vi "dfd_Build Remez Band Parameter from Classical Filter Specs.vi"(6 "fs [Hz]":dbl=1.0 format="%.2f", 7 "filter type":T4(ring), 8 "error in (no error)":errorcluster, 10 "ripple specs":T1={"passband"=0.1, "stopband"=60.0, "dB/linear? (T: dB)"=TRUE}, 11 "freq specs [Hz]":T3) -> (0 "error out":errorcluster, 1 "band ripples":dbl[](array[numeric]), 2 "band parameters":T2[](array[typedef])=[{"band specification"=[{"freq"=0.0, "amplitude"=1.0, "weight"=1.0}, {"freq"=0.2, "amplitude"=1.0, "weight"=1.0}], "ripple constraint"=0.0}, {"band specification"=[{"freq"=0.3, "amplitude"=0.0, "weight"=1.0}, {"freq"=0.5, "amplitude"=0.0, "weight"=1.0}], "ripple constraint"=0.0}])   [LabVIEW 2017, in "NI_DigFilterLicensed.lvlib"]
uses:
  <vilib>/addons/Digital Filter Design/NI_DigFilterLicensed.lvlib
  <vilib>/addons/Digital Filter Design/_Objects.llb/DFD Filter Frequence Specification (Design).ctl
  <vilib>/addons/Digital Filter Design/_Objects.llb/DFD Adv Band Spec.ctl
  <vilib>/addons/Digital Filter Design/_Objects.llb/DFD Filter Ripple Specification (Design).ctl
  <vilib>/addons/Digital Filter Design/NI_DigFilter_Design.lvlib
panel:
  # "freq"
  # "amplitude"
  # "weight"
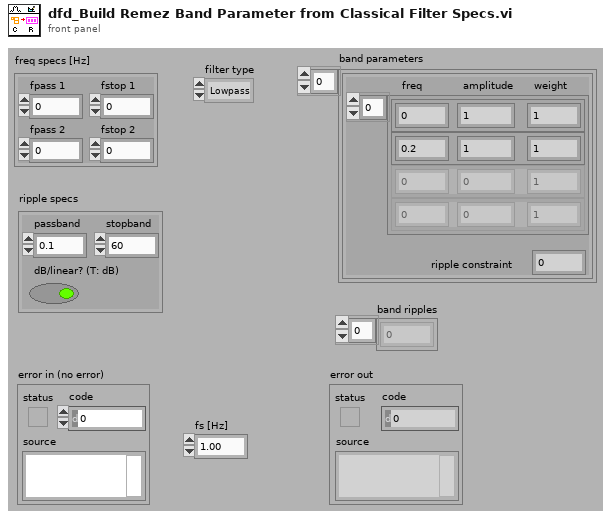
[diagram p1: front panel]
types:
  T1 = typedef "NI_DigFilterLicensed.lvlib/DFD Filter Ripple Specification (Design).ctl" = cluster{"passband":dbl, "stopband":dbl, "dB/linear? (T: dB)":bool}
  T2 = typedef "NI_DigFilterLicensed.lvlib/DFD Adv Band Spec.ctl" = cluster{"band specification":cluster{"freq":dbl, "amplitude":dbl, "weight":dbl}[], "ripple constraint":dbl}
  T3 = typedef "NI_DigFilterLicensed.lvlib/DFD Filter Frequence Specification (Design).ctl" = cluster{"fpass 1":dbl, "fstop 1":dbl, "fpass 2 ":dbl, "fstop 2":dbl}
  T4 = enum16{"Lowpass", "Highpass", "Bandpass", "Bandstop"}
  T5 = cluster{cluster{"fpass 1":dbl, dbl, "stopband":dbl}[], "passband":dbl}
  T6 = cluster{cluster{"fstop 1":dbl, dbl, "passband":dbl}[], "stopband":dbl}
  T7 = cluster{cluster{"fstop 1":dbl, dbl, "passband":dbl}[], "stopband":dbl}[]
  T8 = cluster{cluster{"fpass 1":dbl, dbl, "stopband":dbl}[], "passband":dbl}[]
  T9 = cluster{cluster{"fpass 2 ":dbl, dbl, "stopband":dbl}[], "passband":dbl}
  T10 = cluster{cluster{"fstop 2":dbl, dbl, "passband":dbl}[], "stopband":dbl}
  T11 = cluster{cluster{"fstop 2":dbl, dbl, "passband":dbl}[], "stopband":dbl}[]
  T12 = cluster{cluster{"fpass 2 ":dbl, dbl, "stopband":dbl}[], "passband":dbl}[]
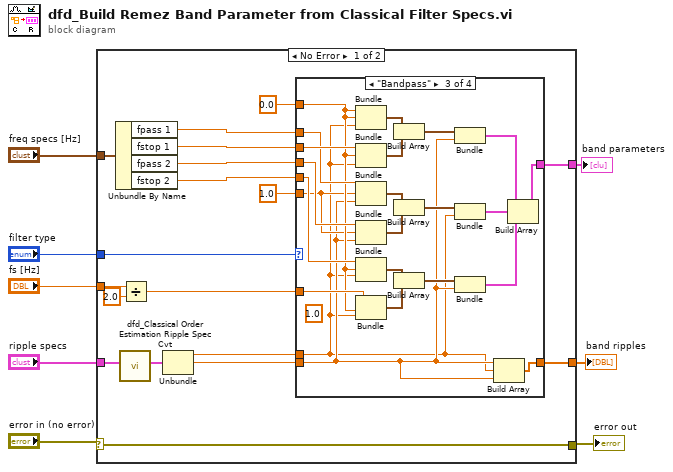
[diagram p0: block diagram]
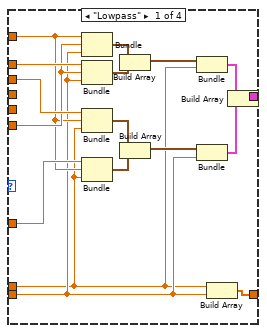
[diagram p2: hidden frame]
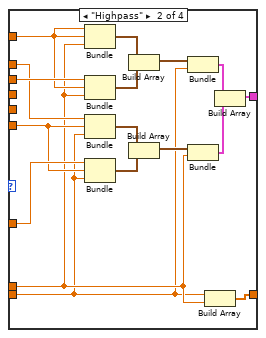
[diagram p3: hidden frame]
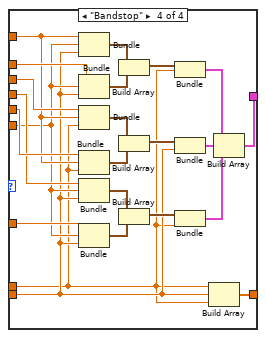
[diagram p4: hidden frame]
diagram:
  n1 = case shown="No Error" "error in (no error)" {
    selector: "error in (no error)" -> [w16 w107]
    tunnel: "filter type" -> [w26 _]
    tunnel: "freq specs [Hz]" -> [w25 _]
    tunnel: [w24 _] -> w6
    tunnel: "fs [Hz]" -> [w19 _]
    tunnel: "ripple specs" -> [w15 _]
    tunnel: [w16 w107] -> w2
    tunnel: [w14 _] -> w1
    frame No Error {
      n2 = Unbundle By Name(w25) -> ("fpass 1"=w23:dbl, "fstop 1"=w22:dbl, "fpass 2"=w21:dbl, "fstop 2"=w20:dbl)
      n3 = call <vilib>:"dfd_Classical Order Estimation Ripple Spec Cvt.vi"("ripple specs"=w15) -> ("ripple specs (linear)"=w13:T1)  [unwired: 10 out]
      n4 = Divide(x=w19, y=2.0) -> (x/y=w17:dbl)
      n5 = Unbundle(w13) -> ("passband"=w12:dbl, "stopband"=w11:dbl)  [unwired: 1 out]
      n6 = case shown="\"Bandpass\"" w26 {
        tunnel: w23 -> [w41 w54 w71 w95]
        tunnel: w22 -> [w35 w55 w72 w94]
        tunnel: w21 -> [_ _ w70 w92]
        tunnel: w20 -> [_ _ w69 w93]
        tunnel: [w34 w51 w67 w90] -> w24
        tunnel: w17 -> [w32 w49 w66 w89]
        tunnel: [w31 w48 w65 w88] -> w14
        tunnel: w12 -> [w27 w45 w61 w84]
        tunnel: w11 -> [w28 w44 w62 w85]
        tunnel: 0.0 -> [w29 w46 w64 w87]
        tunnel: 1.0 -> [w30 w47 w63 w86]
        frame "Lowpass" {
          n7 = Bundle(w29, w30, "stopband"=w28) -> (w43:cluster{dbl, dbl, "stopband":dbl})  [unwired: 1 out]
          n8 = Bundle("fpass 1"=w41, w30, "stopband"=w28) -> (w42:cluster{"fpass 1":dbl, dbl, "stopband":dbl})  [unwired: 1 out]
          n9 = Bundle("fstop 1"=w35, w29, "passband"=w27) -> (w37:cluster{"fstop 1":dbl, dbl, "passband":dbl})  [unwired: 1 out]
          n10 = Bundle(w32, w29, "passband"=w27) -> (w38:cluster{dbl, dbl, "passband":dbl})  [unwired: 1 out]
          n11 = Build Array(w43, w42) -> (w40:cluster{"fpass 1":dbl, dbl, "stopband":dbl}[])
          n12 = Build Array(w37, w38) -> (w39:cluster{"fstop 1":dbl, dbl, "passband":dbl}[])
          n13 = Bundle(w40, "passband"=w27) -> (w33:T5)  [unwired: 1 out]
          n14 = Bundle(w39, "stopband"=w28) -> (w36:T6)  [unwired: 1 out]
          n15 = Build Array(w27, w28) -> (w31:dbl[])
          n16 = Build Array(w33, w36) -> (w34:T7)
        }
        frame "Highpass" {
          n17 = Bundle(w46, w46, "passband"=w45) -> (w56:cluster{dbl, dbl, "passband":dbl})  [unwired: 1 out]
          n18 = Bundle("fstop 1"=w55, w46, "passband"=w45) -> (w52:cluster{"fstop 1":dbl, dbl, "passband":dbl})  [unwired: 1 out]
          n19 = Bundle("fpass 1"=w54, w47, "stopband"=w44) -> (w53:cluster{"fpass 1":dbl, dbl, "stopband":dbl})  [unwired: 1 out]
          n20 = Bundle(w49, w47, "stopband"=w44) -> (w60:cluster{dbl, dbl, "stopband":dbl})  [unwired: 1 out]
          n21 = Build Array(w56, w52) -> (w57:cluster{"fstop 1":dbl, dbl, "passband":dbl}[])
          n22 = Build Array(w53, w60) -> (w59:cluster{"fpass 1":dbl, dbl, "stopband":dbl}[])
          n23 = Bundle(w57, "stopband"=w44) -> (w58:T6)  [unwired: 1 out]
          n24 = Bundle(w59, "passband"=w45) -> (w50:T5)  [unwired: 1 out]
          n25 = Build Array(w44, w45) -> (w48:dbl[])
          n26 = Build Array(w58, w50) -> (w51:T8)
        }
        frame "Bandpass" {
          (unwired) 1.0
          n27 = Bundle(w64, w64, "passband"=w61) -> (w76:cluster{dbl, dbl, "passband":dbl})  [unwired: 1 out]
          n28 = Bundle("fstop 1"=w72, w64, "passband"=w61) -> (w77:cluster{"fstop 1":dbl, dbl, "passband":dbl})  [unwired: 1 out]
          n29 = Bundle("fpass 1"=w71, w63, "stopband"=w62) -> (w81:cluster{"fpass 1":dbl, dbl, "stopband":dbl})  [unwired: 1 out]
          n30 = Bundle("fpass 2"=w70, w63, "stopband"=w62) -> (w80:cluster{"fpass 2 ":dbl, dbl, "stopband":dbl})  [unwired: 1 out]
          n31 = Bundle("fstop 2"=w69, w64, "passband"=w61) -> (w73:cluster{"fstop 2":dbl, dbl, "passband":dbl})  [unwired: 1 out]
          n32 = Bundle(w66, w64, "passband"=w61) -> (w74:cluster{dbl, dbl, "passband":dbl})  [unwired: 1 out]
          n33 = Build Array(w76, w77) -> (w78:cluster{"fstop 1":dbl, dbl, "passband":dbl}[])
          n34 = Build Array(w81, w80) -> (w79:cluster{"fpass 2 ":dbl, dbl, "stopband":dbl}[])
          n35 = Build Array(w73, w74) -> (w75:cluster{"fstop 2":dbl, dbl, "passband":dbl}[])
          n36 = Bundle(w78, "stopband"=w62) -> (w83:T6)  [unwired: 1 out]
          n37 = Bundle(w79, "passband"=w61) -> (w82:T9)  [unwired: 1 out]
          n38 = Bundle(w75, "stopband"=w62) -> (w68:T10)  [unwired: 1 out]
          n39 = Build Array(w62, w61, w62) -> (w65:dbl[])
          n40 = Build Array(w83, w82, w68) -> (w67:T11)
        }
        frame "Bandstop" {
          n41 = Bundle(w87, w86, "stopband"=w85) -> (w103:cluster{dbl, dbl, "stopband":dbl})  [unwired: 1 out]
          n42 = Bundle("fpass 1"=w95, w86, "stopband"=w85) -> (w97:cluster{"fpass 1":dbl, dbl, "stopband":dbl})  [unwired: 1 out]
          n43 = Bundle("fstop 1"=w94, w87, "passband"=w84) -> (w99:cluster{"fstop 1":dbl, dbl, "passband":dbl})  [unwired: 1 out]
          n44 = Bundle("fstop 2"=w93, w87, "passband"=w84) -> (w100:cluster{"fstop 2":dbl, dbl, "passband":dbl})  [unwired: 1 out]
          n45 = Bundle("fpass 2"=w92, w86, "stopband"=w85) -> (w96:cluster{"fpass 2 ":dbl, dbl, "stopband":dbl})  [unwired: 1 out]
          n46 = Bundle(w89, w86, "stopband"=w85) -> (w105:cluster{dbl, dbl, "stopband":dbl})  [unwired: 1 out]
          n47 = Build Array(w103, w97) -> (w102:cluster{"fpass 1":dbl, dbl, "stopband":dbl}[])
          n48 = Build Array(w99, w100) -> (w101:cluster{"fstop 2":dbl, dbl, "passband":dbl}[])
          n49 = Build Array(w96, w105) -> (w104:cluster{"fpass 2 ":dbl, dbl, "stopband":dbl}[])
          n50 = Bundle(w102, "passband"=w84) -> (w98:T5)  [unwired: 1 out]
          n51 = Bundle(w101, "stopband"=w85) -> (w91:T10)  [unwired: 1 out]
          n52 = Bundle(w104, "passband"=w84) -> (w106:T9)  [unwired: 1 out]
          n53 = Build Array(w84, w85, w84) -> (w88:dbl[])
          n54 = Build Array(w98, w91, w106) -> (w90:T12)
        }
      }
    }
    frame Error {
    }
  }
  "band parameters" <- w6
  "error out" <- w2
  "band ripples" <- w1
